vi "Run_VI_Named_specific.vi"(8 "Run VI Named String":string, 10 "Earlier Filenames":path[](array[path]), 11 "Multi Run Row":T1 {"Carrier_2 Q (l/min)" format="%#.2f"; "Row Duration (mins)" format="%#.1f"; "Row No" min=0; "Trace Gas Concentration (%)" min=0.0 format="%#_4f"; "Carrier_1 Q (l/min)" format="%#.4f"; "Start X" format="%#.2f"; "Start Y" format="%#.2f"; "Start Z" format="%#.2f"; "End X" format="%#.2f"; "End Y" format="%#.2f"; "End Z" format="%#.2f"; "Tunnel Speed" format="%#.2f"; "Averaging time (mins)" min=0.0 format="%#.2f"}) -> (0 "Scalable Time (Sec)":dbl format="%.2f", 1 "Fixed Time (Sec)":dbl format="%.2f", 2 "Channel Names":string[](array[string]), 3 "Checks":string[](array[string]), 4 "Error String":string, 5 "Check Meas Setup?":bool, 6 "Check for start NaNs?":bool)   [LabVIEW 2022 SP3]
uses:
  Gen Trav/Traverse_cluster.ctl
  Gen Trav/Spacing.ctl
  Controls/Multi_run_mode.ctl
  Globals/Preference_global.vi
  Globals/Extra_Commands_Global.vi
panel:
  # "X           Y          Z"
  # "Start"
  # "End"
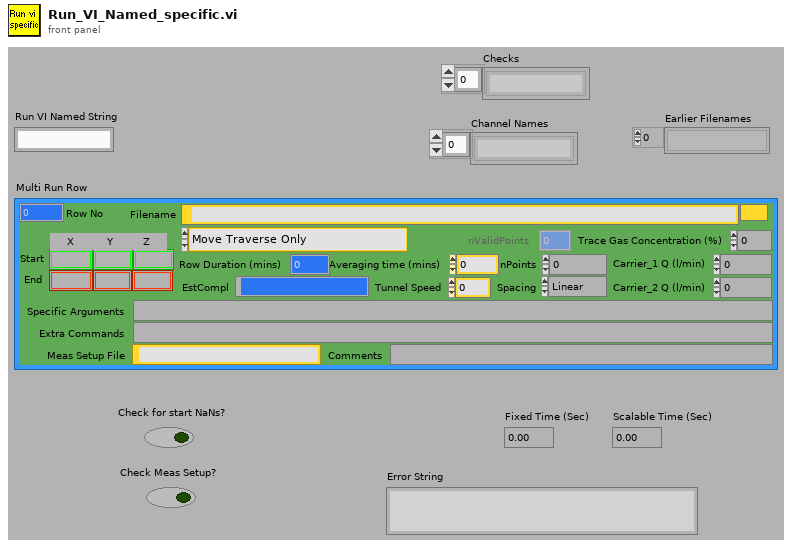
[diagram p1: front panel]
types:
  T1 = typedef "Traverse_cluster.ctl" = cluster{"Start X":sgl, "Start Y":sgl, "Start Z":sgl, "End X":sgl, "End Y":sgl, "End Z":sgl, "nPoints":i32, "Spacing":T2, "Filename":path, "Tunnel Speed":dbl, "Averaging time (mins)":dbl, "Extra Commands":string, "Carrier_1 Q (l/min)":dbl, "Carrier_2 Q (l/min)":dbl, "Trace Gas Concentration (%)":dbl, "Specific Arguments":string, "Comments":string, "Row No":i32, "Row Type Selector":T3, "EstCompl":string, "Row Duration (mins)":dbl, "nValidPoints":i32, "Meas Setup File":string}
  T2 = typedef "Spacing.ctl" = enum16{"Linear", "Log", "Gauss", "Specified", "N/A"}
  T3 = typedef "Multi_run_mode.ctl" = enum16{"Move Traverse Only", "Set Tunnel Speed Only", "Set Source Only", "Set Measurement Conditions", "Single Measurement", "Vertical Profile", "Lateral Profile", "Longitudinal Profile", "Multi-Axis Profile", "Explore Volume", "Auto Calibrate", "Meas Fast FID Bkgnd", "Check Beam Power", "Scanning Valve Measurement", "Run VI Named:", "Set ADAM Ch", "Wait (minutes)", "Send Message", "Synchronize With:", "Fall Back to this Row", "Turn Off Row Repeating", "Traverse 3D Volume", "Blank Row", "Jump to Fall Back Row"}
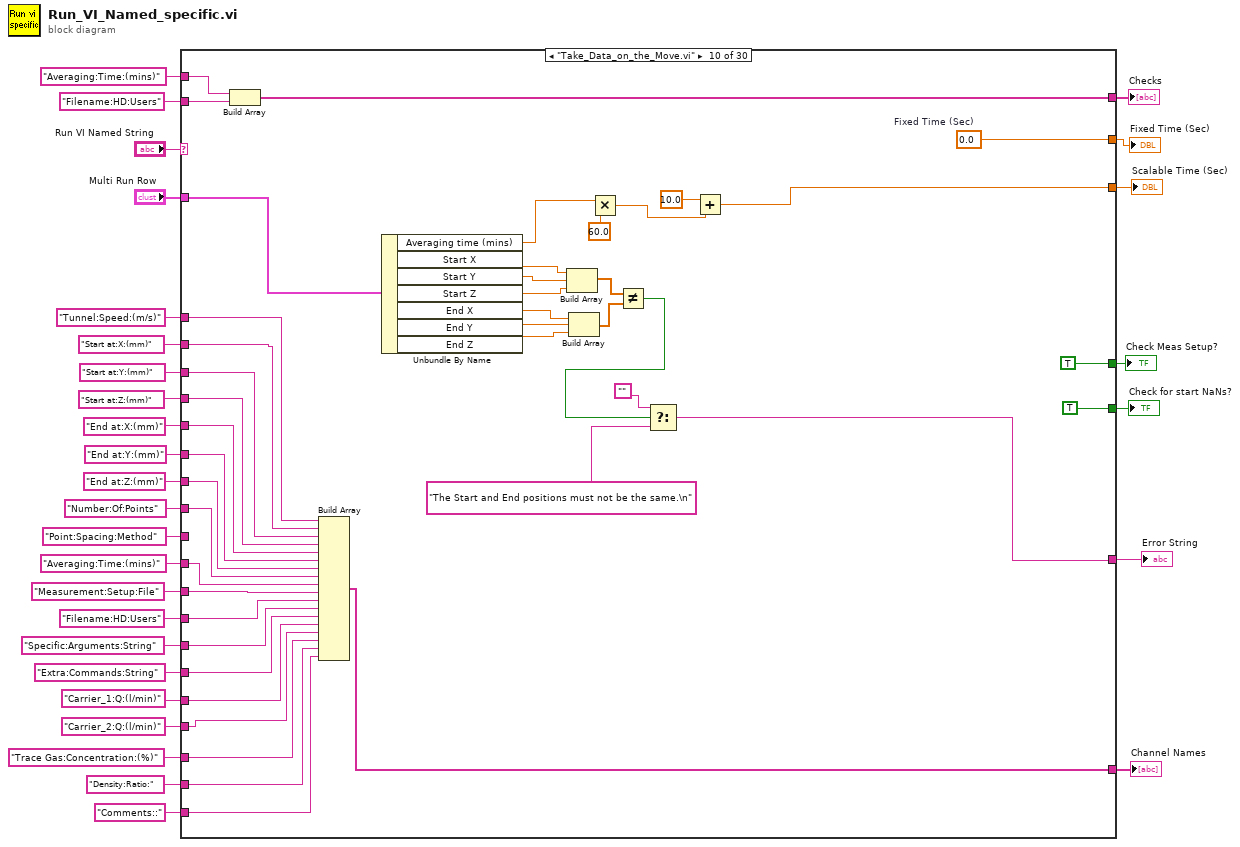
[diagram p0: block diagram]
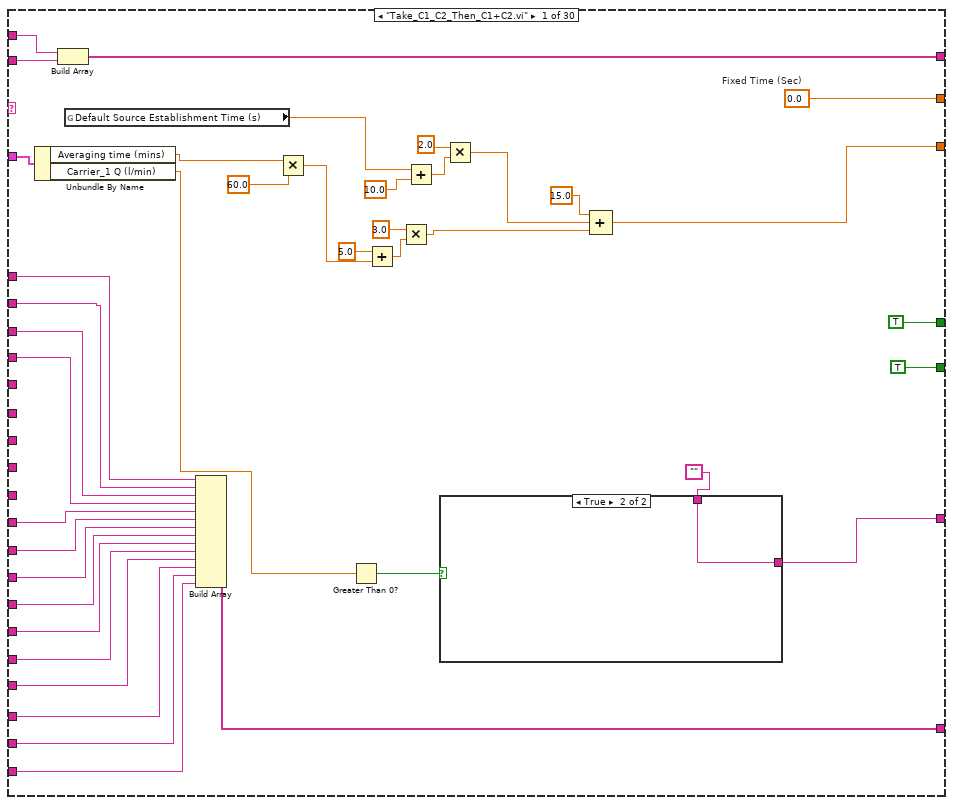
[diagram p2: hidden frame]
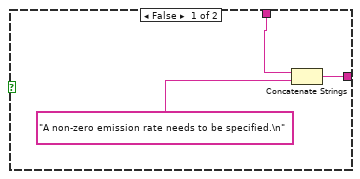
[diagram p3: hidden frame]
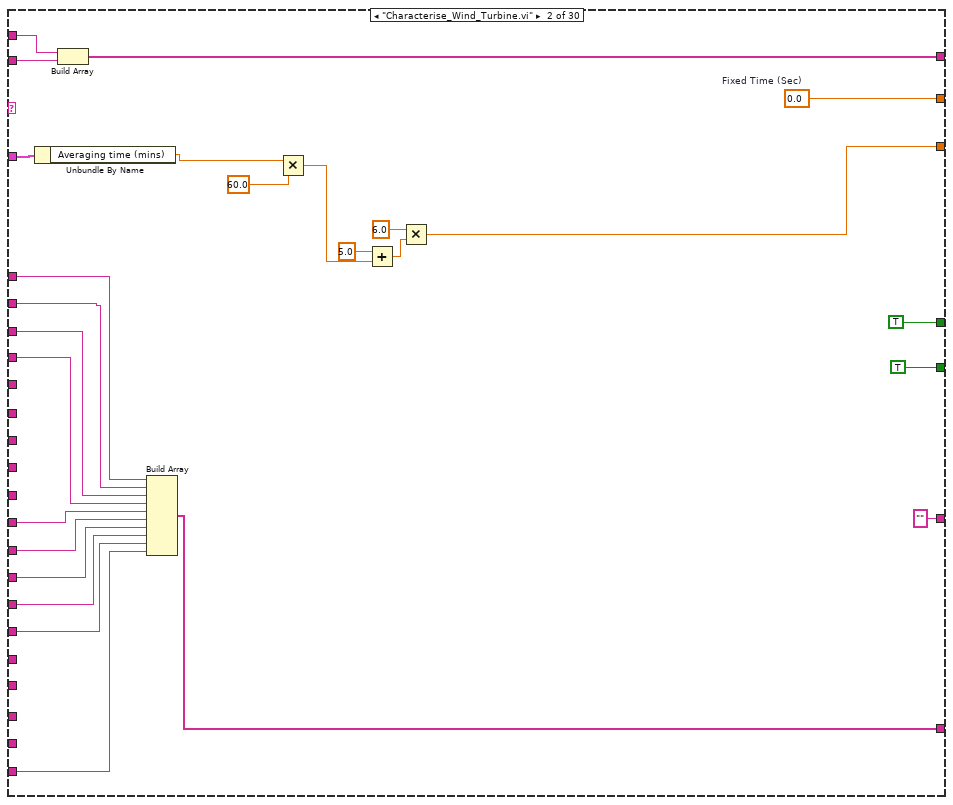
[diagram p4: hidden frame]
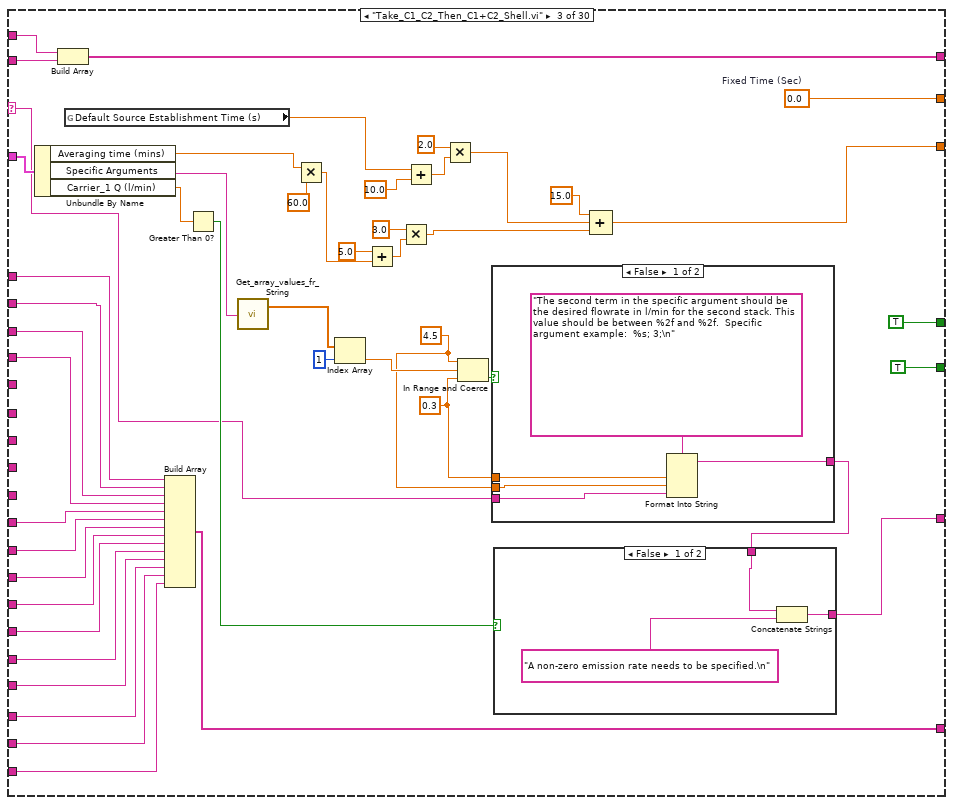
[diagram p5: hidden frame]
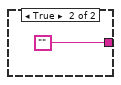
[diagram p7: hidden frame]
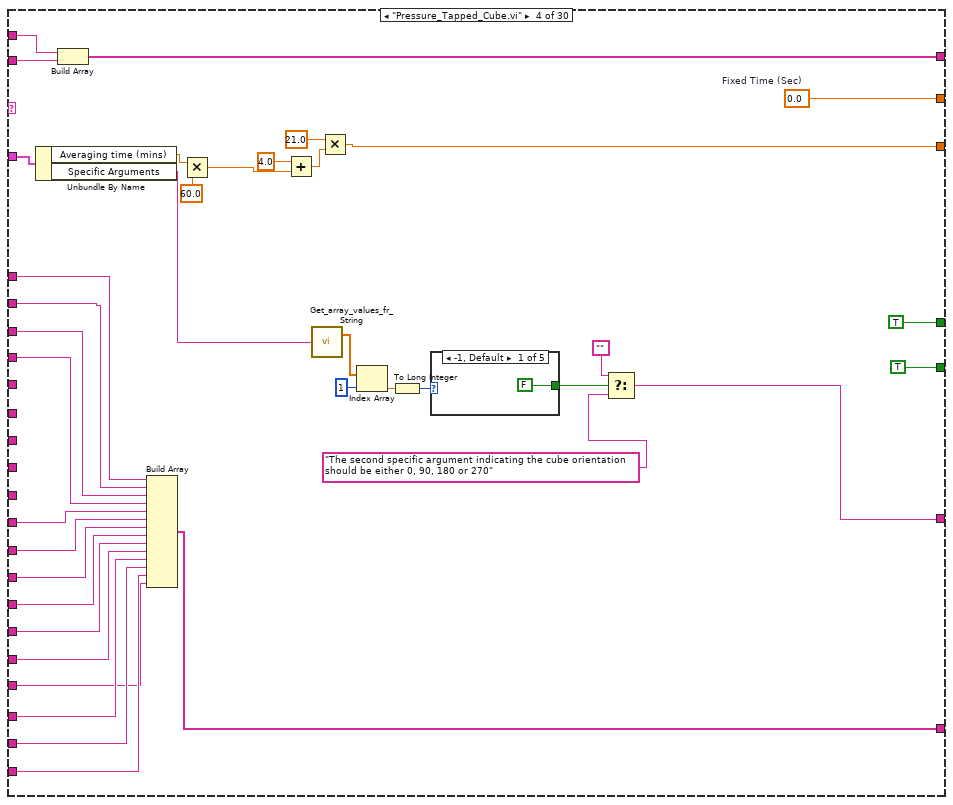
[diagram p8: hidden frame]
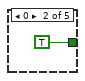
[diagram p9: hidden frame]
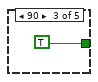
[diagram p10: hidden frame]
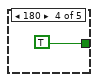
[diagram p11: hidden frame]
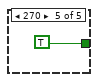
[diagram p12: hidden frame]
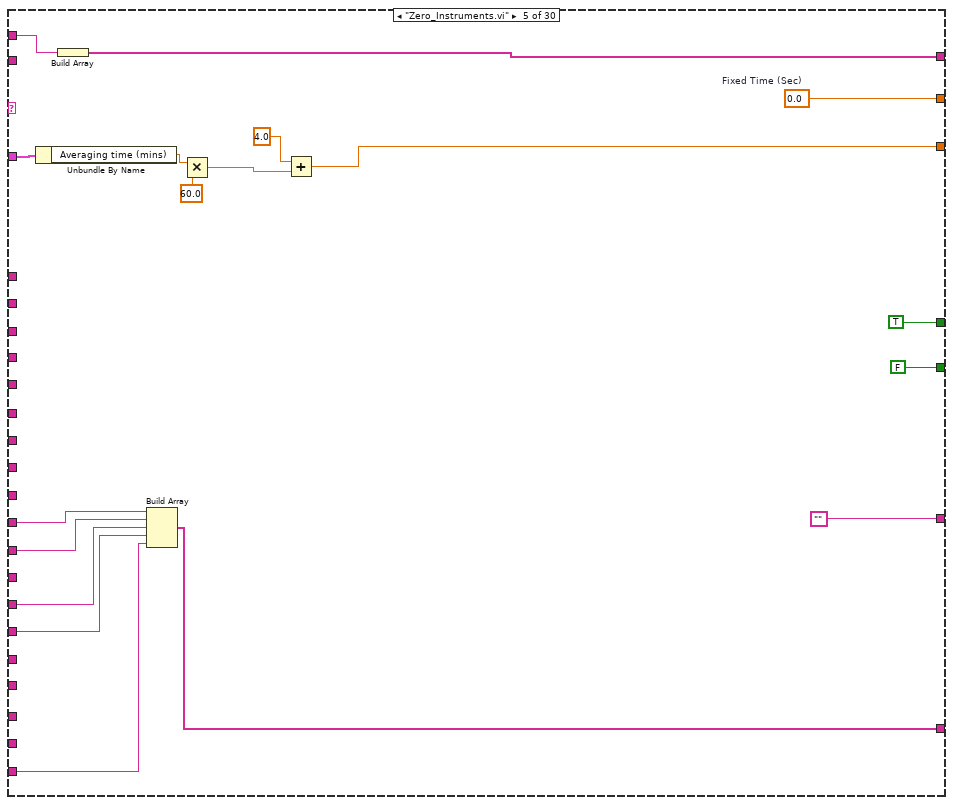
[diagram p13: hidden frame]
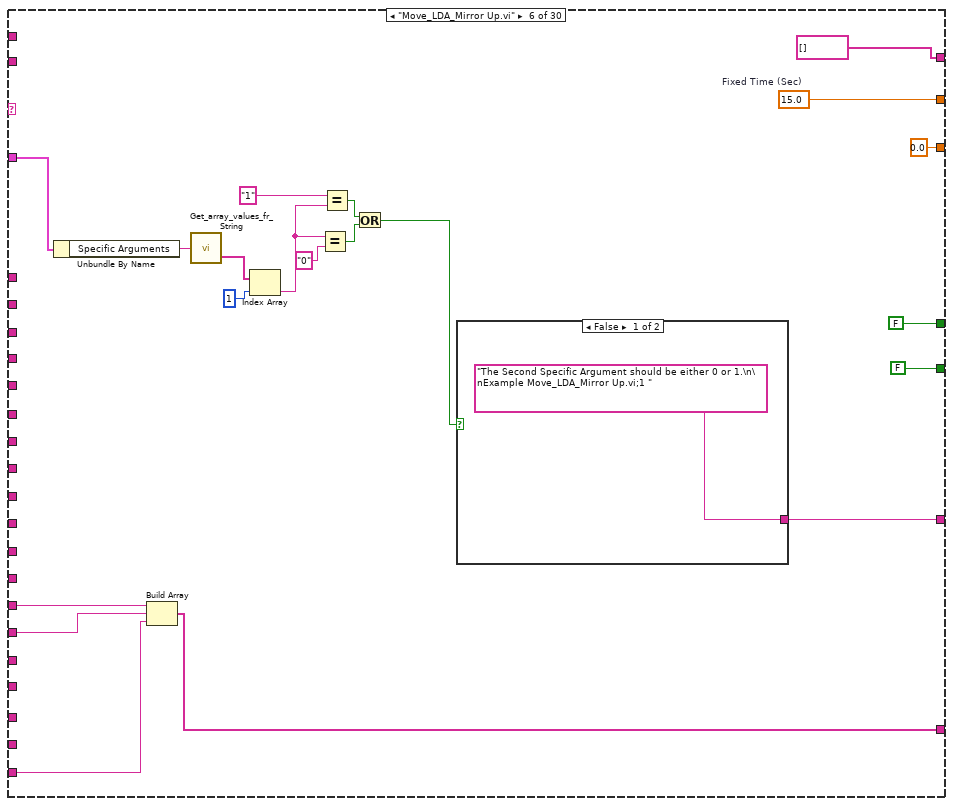
[diagram p14: hidden frame]
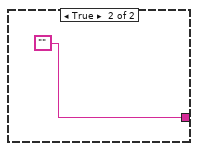
[diagram p15: hidden frame]
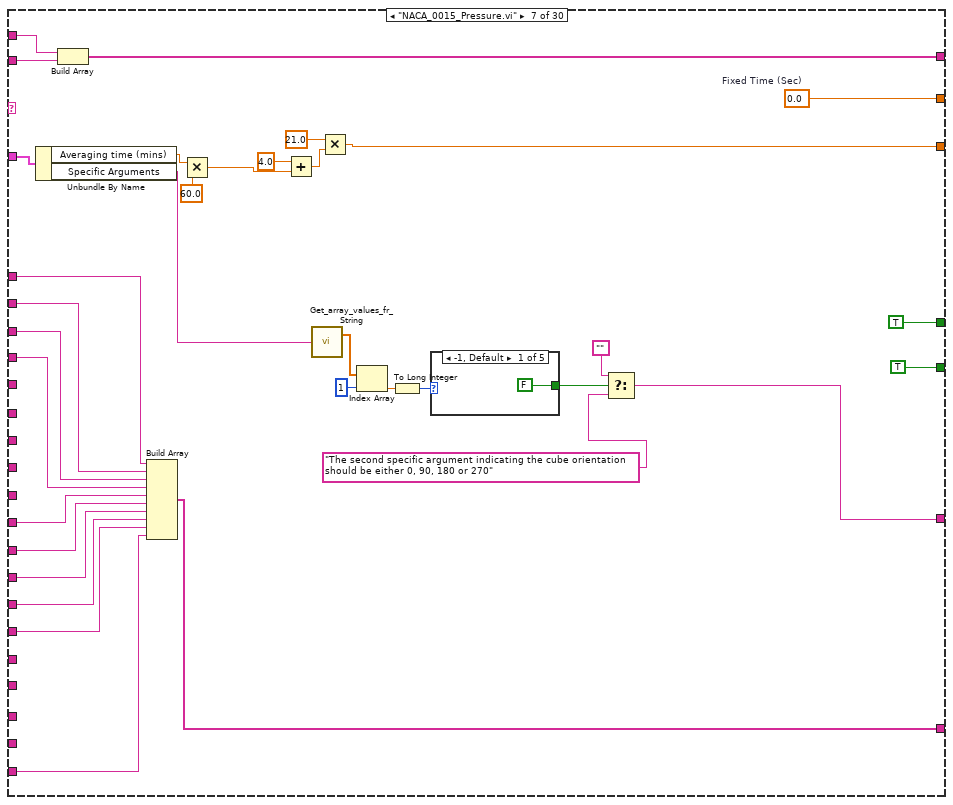
[diagram p16: hidden frame]
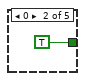
[diagram p17: hidden frame]
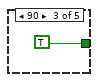
[diagram p18: hidden frame]
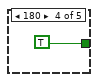
[diagram p19: hidden frame]
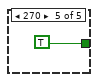
[diagram p20: hidden frame]
diagram:
  n1 = case shown="\"Take_Data_on_the_Move.vi\"" "Run VI Named String" {
    selector: "Run VI Named String" -> [_ _ w103 _ _ _ _ _ _ _ _ _ _ _ _ _ _ _ _ _ _ _ _ _ _ _ _ _ _ _]
    tunnel: "Multi Run Row" -> [w70 w100 w148 w196 w219 w224 w275 w315 w358 w368 _ w422 _ _ _ w500 _ _ w540 _ _ w580 w615 w640 w663 _ _ w741 w769 w801]
    tunnel: [w69 w99 w147 w195 w218 w239 w274 w314 w357 w401 w417 w432 0.0 ("Fixed Time (Sec)") 0.0 ("Fixed Time (Sec)") 5.0 ("Fixed Time (Sec)") 5.0 ("Fixed Time (Sec)") 5.0 ("Fixed Time (Sec)") 5.0 ("Fixed Time (Sec)") 5.0 ("Fixed Time (Sec)") 5.0 ("Fixed Time (Sec)") 5.0 ("Fixed Time (Sec)") 5.0 ("Fixed Time (Sec)") 5.0 ("Fixed Time (Sec)") 5.0 ("Fixed Time (Sec)") 30.0 ("Fixed Time (Sec)") 40.0 ("Fixed Time (Sec)") w709 w733 w768 w800] -> w29
    tunnel: [w55 w76 w133 w169 w202 0.0 ("value") w254 w294 w339 w366 60.0 ("value") 0.0 ("value") 6.0 ("value") 6.0 ("value") 0.0 ("value") 0.0 ("value") 0.0 ("value") 0.0 ("value") w535 0.0 ("value") 0.0 ("value") 0.0 ("value") 0.0 ("value") 0.0 ("value") 270.0 ("value") 0.0 ("value") w710 w740 40.0 ("value") 30.0 ("value")] -> w28
    tunnel: "Averaging:Time:(mins)" ("Label for value") -> [w54 w92 w132 w192 w215 _ w271 w311 w354 w399 w416 _ _ _ _ _ _ _ w543 _ _ _ _ _ _ _ _ _ _ _]
    tunnel: "Filename:HD:Users" ("Label for value") -> [w53 w91 w131 w191 _ _ w270 w310 w353 w398 w415 _ _ _ _ _ _ w524 w541 _ _ _ _ _ _ _ _ _ _ w778]
    tunnel: [TRUE TRUE TRUE TRUE FALSE FALSE TRUE TRUE FALSE TRUE TRUE FALSE FALSE FALSE FALSE FALSE FALSE FALSE FALSE FALSE FALSE FALSE FALSE FALSE FALSE FALSE FALSE FALSE TRUE TRUE] -> w25
    tunnel: [TRUE TRUE TRUE TRUE TRUE FALSE TRUE TRUE TRUE TRUE TRUE FALSE FALSE FALSE FALSE FALSE FALSE TRUE TRUE FALSE FALSE FALSE FALSE FALSE FALSE FALSE FALSE TRUE FALSE TRUE] -> w24
    tunnel: [w50 w88 w128 w188 w212 string[] [] w267 w307 w350 w395 w412 string[] [] string[] [] string[] [] string[] [] string[] [] string[] [] string[] [] w542 string[] [] string[] [] string[] [] string[] [] string[] [] string[] [] string[] [] string[] [] string[] [] string[] [] w777] -> w23
    tunnel: "Tunnel:Speed:(m/s)" ("Label for value") -> [w49 w87 w127 w187 _ _ w244 w284 _ w394 _ w423 w447 w473 _ _ _ _ _ _ _ _ _ _ _ _ _ w720 _ _]
    tunnel: "Start at:X:(mm)" ("Label for value") -> [w48 w86 w126 w186 _ _ w243 w283 _ w393 w411 _ w456 w477 _ _ w515 _ _ _ _ _ w614 w647 w671 w691 _ _ w765 w797]
    tunnel: "Start at:Y:(mm)" ("Label for value") -> [w47 w85 w125 w185 _ _ w242 w282 _ w392 w410 _ w455 w476 _ _ _ _ _ _ _ _ w613 _ _ w694 _ _ w764 w796]
    tunnel: "Start at:Z:(mm)" ("Label for value") -> [w46 w84 w124 w184 _ _ w266 w306 _ w391 w409 _ w454 w475 _ _ _ _ _ _ _ _ w612 _ _ _ _ _ w763 w795]
    tunnel: "Averaging:Time:(mins)" ("Label for value") -> [w45 w83 w123 w183 w211 _ w265 w305 w335 w390 _ _ w446 w472 _ _ _ _ w545 _ _ _ _ _ _ _ _ w729 _ _]
    tunnel: "Measurement:Setup:File" ("Label for value") -> [w44 w82 w122 w182 w210 _ w264 w304 w349 w389 w408 _ w442 w468 _ _ _ w526 w546 _ _ _ w609 w644 w667 w695 _ w730 _ w779]
    tunnel: "Filename:HD:Users" ("Label for value") -> [w43 w81 w121 w181 _ _ w263 w303 w348 w388 _ _ w448 w474 _ _ _ _ w544 _ _ w581 w610 w645 _ _ _ w731 _ w776]
    tunnel: "Specific:Arguments:String" ("Label for value") -> [w42 w80 w120 w180 w209 w235 w262 w302 w347 w387 w407 w429 w441 w467 w491 w511 w521 w532 w552 w562 w572 w588 w611 w646 w668 w696 w717 w732 w756 w775]
    tunnel: "Extra:Commands:String" ("Label for value") -> [w41 w79 w119 w179 w208 w231 w261 w301 w346 w386 w406 w428 w440 w466 w490 w510 _ _ w551 w561 w571 w587 w622 w655 w669 w697 w716 w745 w757 w791]
    tunnel: "Carrier_1:Q:(l/min)" ("Label for value") -> [w31 _ w101 w178 _ _ _ _ _ w385 _ _ w445 w471 _ _ _ _ _ _ _ _ _ _ _ _ _ _ _ _]
    tunnel: "Trace Gas:Concentration:(%)" ("Label for value") -> [w40 _ w118 w177 _ _ _ _ _ w361 _ _ w444 w470 _ _ _ _ _ _ _ _ _ _ _ _ _ _ _ _]
    tunnel: "Density:Ratio:" ("Label for value") -> [w39 _ w117 w176 _ _ _ _ _ w384 _ _ w443 w469 _ _ _ _ _ _ _ _ _ _ _ _ _ _ _ _]
    tunnel: "Comments::" ("Label for value") -> [w38 w78 w116 w175 w204 w232 w260 w300 w345 w383 w405 w427 w439 w465 w489 w509 w520 w531 w550 w560 w570 w586 w621 w654 w670 w698 w715 w744 w760 w792]
    tunnel: [w37 w77 w115 w174 w207 w236 w259 w299 w344 w382 w404 w426 w438 w464 w488 w508 w519 w530 w549 w559 w569 w585 w620 w653 w675 w703 w714 w743 w762 w794] -> w10
    tunnel: [w35 "" ("Error Comments") w104 w160 "" w220 w245 w285 w337 w365 "" w418 "" "" "" w494 "" "" "" "" "" w576 w599 "" w660 "" "" w735 w759 w780] -> w3
    tunnel: "End at:X:(mm)" ("Label for value") -> [_ _ _ _ _ _ _ _ _ w364 _ _ w453 _ _ _ _ _ _ _ _ _ _ _ _ w693 _ _ _ w793]
    tunnel: "End at:Y:(mm)" ("Label for value") -> [_ _ _ _ _ _ _ _ _ w363 _ _ w452 _ _ _ _ _ _ _ _ _ _ _ _ w692 _ _ _ _]
    tunnel: "End at:Z:(mm)" ("Label for value") -> [_ _ _ _ _ _ _ _ _ w362 _ _ w451 _ _ _ _ _ _ _ _ _ _ _ _ _ _ _ _ _]
    tunnel: "Number:Of:Points" ("Label for value") -> [_ _ _ _ _ _ _ w281 w336 w359 _ _ w450 _ _ _ _ _ _ _ _ _ _ _ _ _ _ _ _ _]
    tunnel: "Point:Spacing:Method" ("Label for value") -> [_ _ _ _ _ _ _ _ w334 _ _ _ w449 _ _ _ _ _ _ _ _ _ _ _ _ _ _ _ _ _]
    tunnel: "Carrier_2:Q:(l/min)" ("Label for value") -> [w32 _ w102 w159 _ _ _ _ _ w360 _ _ w437 w463 _ _ _ _ _ _ _ _ _ _ _ _ _ _ _ _]
    frame "Take_C1_C2_Then_C1+C2.vi" {
      w69 = 0.0  # Fixed Time (Sec)
      n2 = Unbundle By Name(w70) -> ("Averaging time (mins)"=w58:dbl, "Carrier_1 Q (l/min)"=w34:dbl)
      n3 = Build Array(w54, w53) -> (w50:string[])
      n4 = global read "Preference_global.vi" "Default Source Establishment Time (s)"() -> (w59:dbl)
      n5 = Build Array(w49, w48, w47, w46, w45, w44, w43, w42, w41, w31, w32, w40, w39, w38) -> (w37:string[])
      n6 = Multiply(x=w58, y=60.0) -> (x*y=w56:dbl)
      n7 = Greater Than 0?(x=w34) -> (x > 0?=w33:bool)
      n8 = Add(x=5.0, y=w56) -> (x+y=w62:dbl)
      n9 = Multiply(x=3.0, y=w62) -> (x*y=w66:dbl)
      n10 = Add(x=w59, y=10.0) -> (x+y=w64:dbl)
      n11 = case shown="True" w33 {
        tunnel: "" -> [w72 w74]
        tunnel: [w71 w74] -> w35
        frame False {
          n12 = Concatenate Strings(w72, "A non-zero emission rate needs to be specified.\n") -> (w71:string)
        }
        frame True {
        }
      }
      n13 = Multiply(x=2.0, y=w64) -> (x*y=w67:dbl)
      n14 = Compound Arithmetic op=ADD(15.0 ("value"), w67, w66) -> (w55:dbl)
    }
    frame "Characterise_Wind_Turbine.vi" {
      w99 = 0.0  # Fixed Time (Sec)
      n15 = Unbundle By Name(w100) -> ("Averaging time (mins)"=w95:dbl)
      n16 = Build Array(w92, w91) -> (w88:string[])
      n17 = Build Array(w87, w86, w85, w84, w83, w82, w81, w80, w79, w78) -> (w77:string[])
      n18 = Multiply(x=w95, y=60.0) -> (x*y=w93:dbl)
      n19 = Add(x=5.0, y=w93) -> (x+y=w98:dbl)
      n20 = Multiply(x=6.0, y=w98) -> (x*y=w76:dbl)
    }
    frame "Take_C1_C2_Then_C1+C2_Shell.vi" {
      w108 = 4.5 ("upper limit")
      w109 = 0.3 ("lower limit")
      w147 = 0.0  # Fixed Time (Sec)
      n21 = Unbundle By Name(w148) -> ("Averaging time (mins)"=w136:dbl, "Specific Arguments"=w112:string, "Carrier_1 Q (l/min)"=w107:dbl)
      n22 = Build Array(w132, w131) -> (w128:string[])
      n23 = global read "Preference_global.vi" "Default Source Establishment Time (s)"() -> (w137:dbl)
      n24 = Build Array(w127, w126, w125, w124, w123, w122, w121, w120, w119, w101, w102, w118, w117, w116) -> (w115:string[])
      n25 = Greater Than 0?(x=w107) -> (x > 0?=w106:bool)
      n26 = call "Get_array_values_fr_String.vi"("String Value"=w112) -> ("Numeric Array"=w114:dbl[])  [unwired: 1 out]
      n27 = Multiply(x=w136, y=60.0) -> (x*y=w134:dbl)
      n28 = Index Array(array=w114, index=1) -> (element=w111:dbl)
      n29 = Add(x=5.0, y=w134) -> (x+y=w140:dbl)
      n30 = Multiply(x=3.0, y=w140) -> (x*y=w144:dbl)
      n31 = Add(x=w137, y=10.0) -> (x+y=w142:dbl)
      n32 = Multiply(x=2.0, y=w142) -> (x*y=w145:dbl)
      n33 = In Range and Coerce(upper limit=w108, x=w111, lower limit=w109) -> (In Range?=w110:bool)  [unwired: 1 out]
      n34 = case shown="False" w110 {
        tunnel: [w153 ""] -> w105
        tunnel: w103 -> [w157 _]
        tunnel: w109 -> [w156 _]
        tunnel: w108 -> [w155 _]
        frame False {
          n35 = Format Into String(format string="The second term in the specific argument should be the desired flowrate in l/min for the second stack. This value should be between %2f and %2f.  Specific argument example:  %s; 3;\n", w156, w155, w157) -> (resulting string=w153:string)  [unwired: 2 in, 1 out]
        }
        frame True {
        }
      }
      n36 = case shown="False" w106 {
        tunnel: w105 -> [w150 w152]
        tunnel: [w149 w152] -> w104
        frame False {
          n37 = Concatenate Strings(w150, "A non-zero emission rate needs to be specified.\n") -> (w149:string)
        }
        frame True {
        }
      }
      n38 = Compound Arithmetic op=ADD(15.0 ("value"), w145, w144) -> (w133:dbl)
    }
    frame "Pressure_Tapped_Cube.vi" {
      w195 = 0.0  # Fixed Time (Sec)
      n39 = Unbundle By Name(w196) -> ("Averaging time (mins)"=w194:dbl, "Specific Arguments"=w161:string)
      n40 = Build Array(w192, w191) -> (w188:string[])
      n41 = Build Array(w187, w186, w185, w184, w183, w182, w181, w180, w179, w178, w177, w176, w175, w159) -> (w174:string[])
      n42 = Multiply(x=w194, y=60.0) -> (x*y=w170:dbl)
      n43 = Add(x=4.0, y=w170) -> (x+y=w173:dbl)
      n44 = call "Get_array_values_fr_String.vi"("String Value"=w161) -> ("Numeric Array"=w163:dbl[])  [unwired: 1 out]
      n45 = Multiply(x=21.0, y=w173) -> (x*y=w169:dbl)
      n46 = Index Array(array=w163, index=1) -> (element=w164:dbl)
      n47 = To Long Integer(number=w164) -> (32bit integer=w165:i32)
      n48 = case shown="-1, Default" w165 {
        tunnel: [FALSE TRUE TRUE TRUE TRUE] -> w168
        frame -1, Default {
        }
        frame 0 {
        }
        frame 90 {
        }
        frame 180 {
        }
        frame 270 {
        }
      }
      n49 = Select(t="", s=w168, f="The second specific argument indicating the cube orientation should be either 0, 90, 180 or 270") -> (s? t:f=w160:string)
    }
    frame "Zero_Instruments.vi" {
      w218 = 0.0  # Fixed Time (Sec)
      n50 = Unbundle By Name(w219) -> ("Averaging time (mins)"=w217:dbl)
      n51 = Build Array(w215) -> (w212:string[])
      n52 = Build Array(w211, w210, w209, w208, w204) -> (w207:string[])
      n53 = Multiply(x=w217, y=60.0) -> (x*y=w205:dbl)
      n54 = Add(x=4.0, y=w205) -> (x+y=w202:dbl)
    }
    frame "Move_LDA_Mirror Up.vi" {
      w239 = 15.0  # Fixed Time (Sec)
      n55 = Unbundle By Name(w224) -> ("Specific Arguments"=w225:string)
      n56 = Build Array(w235, w231, w232) -> (w236:string[])
      n57 = call "Get_array_values_fr_String.vi"("String Value"=w225) -> ("String array"=w227:string[])  [unwired: 1 out]
      n58 = Index Array(array=w227, index=1) -> (element=w229:string)
      n59 = Equal?(x=w229, y="0") -> (x = y?=w222:bool)
      n60 = Equal?(x="1" ("String to match"), y=w229) -> (x = y?=w223:bool)
      n61 = Or(x=w223, y=w222) -> (x .or. y?=w221:bool)
      n62 = case shown="False" w221 {
        tunnel: ["The Second Specific Argument should be either 0 or 1.\n\nExample Move_LDA_Mirror Up.vi;1 " ""] -> w220
        frame False {
        }
        frame True {
        }
      }
    }
    frame "NACA_0015_Pressure.vi" {
      w274 = 0.0  # Fixed Time (Sec)
      n63 = Unbundle By Name(w275) -> ("Averaging time (mins)"=w273:dbl, "Specific Arguments"=w246:string)
      n64 = Build Array(w271, w270) -> (w267:string[])
      n65 = Build Array(w244, w243, w242, w266, w265, w264, w263, w262, w261, w260) -> (w259:string[])
      n66 = Multiply(x=w273, y=60.0) -> (x*y=w255:dbl)
      n67 = Add(x=4.0, y=w255) -> (x+y=w258:dbl)
      n68 = call "Get_array_values_fr_String.vi"("String Value"=w246) -> ("Numeric Array"=w248:dbl[])  [unwired: 1 out]
      n69 = Multiply(x=21.0, y=w258) -> (x*y=w254:dbl)
      n70 = Index Array(array=w248, index=1) -> (element=w249:dbl)
      n71 = To Long Integer(number=w249) -> (32bit integer=w250:i32)
      n72 = case shown="-1, Default" w250 {
        tunnel: [FALSE TRUE TRUE TRUE TRUE] -> w253
        frame -1, Default {
        }
        frame 0 {
        }
        frame 90 {
        }
        frame 180 {
        }
        frame 270 {
        }
      }
      n73 = Select(t="", s=w253, f="The second specific argument indicating the cube orientation should be either 0, 90, 180 or 270") -> (s? t:f=w245:string)
    }
    frame "NACA_0015_Pressure_with_profile.vi" {
      w314 = 0.0  # Fixed Time (Sec)
      n74 = Unbundle By Name(w315) -> ("Averaging time (mins)"=w313:dbl, "Specific Arguments"=w286:string)
      n75 = Build Array(w311, w310) -> (w307:string[])
      n76 = Build Array(w284, w283, w282, w306, w281, w305, w304, w303, w302, w301, w300) -> (w299:string[])
      n77 = Multiply(x=w313, y=60.0) -> (x*y=w295:dbl)
      n78 = Add(x=4.0, y=w295) -> (x+y=w298:dbl)
      n79 = call "Get_array_values_fr_String.vi"("String Value"=w286) -> ("Numeric Array"=w288:dbl[])  [unwired: 1 out]
      n80 = Multiply(x=21.0, y=w298) -> (x*y=w294:dbl)
      n81 = Index Array(array=w288, index=1) -> (element=w289:dbl)
      n82 = To Long Integer(number=w289) -> (32bit integer=w290:i32)
      n83 = case shown="-1, Default" w290 {
        tunnel: [FALSE TRUE TRUE TRUE TRUE] -> w293
        frame -1, Default {
        }
        frame 0 {
        }
        frame 90 {
        }
        frame 180 {
        }
        frame 270 {
        }
      }
      n84 = Select(t="", s=w293, f="The second specific argument indicating the cube orientation should be either 0, 90, 180 or 270") -> (s? t:f=w285:string)
    }
    frame "Measure_Synthetic_Jet.vi" {
      w357 = 0.0  # Fixed Time (Sec)
      n85 = Unbundle By Name(w358) -> ("Averaging time (mins)"=w356:dbl, "Specific Arguments"=w338:string)
      n86 = Build Array(w354, w353) -> (w350:string[])
      n87 = Build Array(w336, w334, w335, w349, w348, w347, w346, w345) -> (w344:string[])
      n88 = Multiply(x=w356, y=60.0) -> (x*y=w340:dbl)
      n89 = Add(x=4.0, y=w340) -> (x+y=w343:dbl)
      n90 = call "Get_array_values_fr_String.vi"("String Value"=w338) -> ("String array"=w333:string[])  [unwired: 1 out]
      n91 = Multiply(x=21.0, y=w343) -> (x*y=w339:dbl)
      n92 = Index Array(array=w333, index #1=1 ("index")) -> (element #1=w328:string, element #2=w326:string, element #3=w325:string, element #4=w322:string)  [unwired: 3 in]
      n93 = Empty String/Path?(string/path=w322) -> (empty?=w321:bool)
      n94 = Empty String/Path?(string/path=w326) -> (empty?=w323:bool)
      n95 = Empty String/Path?(string/path=w328) -> (empty?=w327:bool)
      n96 = Empty String/Path?(string/path=w325) -> (empty?=w324:bool)
      n97 = Compound Arithmetic op=OR(w327, w323, w324, w321) -> (w331:bool)
      n98 = Select(t="The second, third and fourth specific argument indicate the min frequency, max frequency, the number of bins to use in the phase average and the target amplitude.  Set the target optimisation target value to -1 if you do not want any optimisation. Example: Measure_Synthetic_Jet.vi; 100; 1000; 50; 0.02", s=w331, f="") -> (s? t:f=w337:string)
    }
    frame "Take_Data_on_the_Move.vi" {
      w401 = 0.0  # Fixed Time (Sec)
      n99 = Build Array(w399, w398) -> (w395:string[])
      n100 = Build Array(w394, w393, w392, w391, w364, w363, w362, w359, w390, w389, w388, w387, w386, w385, w360, w361, w384, w383) -> (w382:string[])
      n101 = Unbundle By Name(w368) -> ("Averaging time (mins)"=w367:dbl, "Start X"=w369:sgl, "Start Y"=w370:sgl, "Start Z"=w371:sgl, "End X"=w372:sgl, "End Y"=w373:sgl, "End Z"=w374:sgl)
      n102 = Build Array(w369, w370, w371) -> (w376:sgl[])
      n103 = Build Array(w372, w373, w374) -> (w375:sgl[])
      n104 = Multiply(x=w367, y=60.0) -> (x*y=w380:dbl)
      n105 = Not Equal?(x=w376, y=w375) -> (x != y?=w379:bool)
      n106 = Select(t="", s=w379, f="The Start and End positions must not be the same.\n" ("Format String")) -> (s? t:f=w365:string)
      n107 = Add(x=10.0, y=w380) -> (x+y=w366:dbl)
    }
    frame "Check_FID_Response.vi" {
      w417 = 0.0  # Fixed Time (Sec)
      n108 = Build Array(w416, w415) -> (w412:string[])
      n109 = Build Array(w411, w410, w409, w408, w407, w406, w405) -> (w404:string[])
    }
    frame "Return_EnFlo_Tunnel_to_Neutral.vi" {
      w419 = 0.4 ("y")
      w432 = 6000.0  # Fixed Time (Sec)
      n110 = Unbundle By Name(w422) -> ("Tunnel Speed"=w421:dbl)
      n111 = Build Array(w423, w429, w428, w427) -> (w426:string[])
      n112 = Greater?(x=w421, y=w419) -> (0:w420:bool)
      n113 = case shown="False" w420 {
        tunnel: w419 -> [w435 _]
        tunnel: [w433 ""] -> w418
        frame False {
          n114 = Format Into String(format string="The Tunnel speed must be greater than %.1f", w435) -> (resulting string=w433:string)  [unwired: 2 in, 1 out]
        }
        frame True {
        }
      }
    }
    frame "No Match", Default {
      n115 = Build Array(w456, w455, w454, w453, w452, w451, w450, w449, w448, w447, w446, w440, w441, w445, w444, w443, w439, w442, w437) -> (w438:string[])
    }
    frame "Measurement on Remote PC.vi" {
      n116 = Build Array(w477, w476, w475, w474, w473, w472, w466, w467, w471, w470, w469, w465, w468, w463) -> (w464:string[])
    }
    frame "Set_Wind_Turbine_Speed.vi" {
      n117 = Build Array(w491, w490, w489) -> (w488:string[])
    }
    frame "Wait till chilled water below.vi" {
      n118 = Unbundle By Name(w500) -> ("Specific Arguments"=w499:string)
      n119 = Build Array(w511, w510, w509) -> (w508:string[])
      n120 = call "Get_array_values_fr_String.vi"("String Value"=w499) -> ("Numeric Array"=w502:dbl[])  [unwired: 1 out]
      n121 = Index Array(array=w502, index=1) -> (element=w498:dbl)
      n122 = In Range and Coerce(upper limit=25.0, x=w498, lower limit=4.0) -> (In Range?=w495:bool)  [unwired: 1 out]
      n123 = Select(t="", s=w495, f="The second specific argument setting  the chilled water temperature below which the run can continue should be in the range of 4 to 25 degC.") -> (s? t:f=w494:string)
    }
    frame "CPP-MoveTT.vi" {
      # "Desired angle can now be held in X; previously passed after semicolon in Specific Arguments"
      n124 = Build Array(w515, w521, w520) -> (w519:string[])
    }
    frame "ESC Run VI Named.vi" {
      n125 = Build Array(w524, w526, w532, w531) -> (w530:string[])
    }
    frame "Capture_Flow_Vis.vi" {
      n126 = Build Array(w543, w541) -> (w542:string[])
      n127 = Unbundle By Name(w540) -> ("Averaging time (mins)"=w539:dbl)
      n128 = Build Array(w545, w546, w544, w552, w551, w550) -> (w549:string[])
      n129 = Multiply(x=60.0, y=w539) -> (x*y=w537:dbl)
      n130 = Add(x=w537, y=60.0) -> (x+y=w535:dbl)
    }
    frame "Shut_Down_A_Tunnel.vi", "Shut_down_EnFlo_Tunnel.vi" {
      n131 = Build Array(w562, w561, w560) -> (w559:string[])
    }
    frame "Post Process Files in MultiRun.vi", "Shut_Down_Aero_Tunnel.vi" {
      n132 = Build Array(w572, w571, w570) -> (w569:string[])
    }
    frame "Update_Inlet_Temp_Profile.vi" {
      n133 = Unbundle By Name(w580) -> ("Filename"=w575:path)
      n134 = Build Array(w581, w588, w587, w586) -> (w585:string[])
      n135 = Search 1D Array(1D array="Earlier Filenames", element=w575) -> (index of element=w578:i32)  [unwired: 1 in]
      n136 = case shown="0, Default" w578 {
        tunnel: w575 -> [_ w597]
        tunnel: [TRUE ("exists?") w596] -> w577
        frame 0, Default {
        }
        frame -1 {
          n137 = call "Does_file_exist_(simple).vi"("Pathname"=w597) -> ("exists?"=w596:bool)
        }
      }
      n138 = case shown="False" w577 {
        tunnel: [w591 ""] -> w576
        tunnel: w575 -> [w593 _]
        frame False {
          n139 = Format Into String(format string="Cannot find Filename%s", w593) -> (resulting string=w591:string)  [unwired: 2 in, 1 out]
        }
        frame True {
        }
      }
    }
    frame "Datum_Image_Calibration.vi" {
      n140 = Unbundle By Name(w615) -> ("Filename"=w606:path, "Specific Arguments"=w604:string)
      n141 = Build Array(w614, w613, w612, w609, w610, w611, w622, w621) -> (w620:string[])
      n142 = disable-structure shown="TARGET_TYPE==Windows" {
        disable-tunnel: [w625 _] -> w598
        frame condition #0 (active) {
          n143 = call "Get_Available_Cameras.vi"() -> ("Cameras"=w625:string[])  [unwired: 2 in, 1 out]
        }
        frame condition #1 {
        }
      }
      n144 = call "Get_array_values_fr_String.vi"("String Value"=w604) -> ("String array"=w603:string[])  [unwired: 1 out]
      n145 = call "Current_Filepath.vi"("Short_Name"="Cal" ("Data Type"), "Filename in"=w606, "Data Type"="Calibrations") -> ("Filename Out"=w605:path)  [unwired: 1 in, 1 out]
      n146 = Index Array(array=w603, index=2) -> (element=w600:string)
      n147 = call "Does_file_exist_(simple).vi"("Pathname"=w605) -> ("exists?"=w616:bool)
      n148 = case shown="False" w616 {
        tunnel: w605 -> [w638 _]
        frame False {
          n149 = call "Write Characters with check.vi"("String to Write"="Created so that multirun checker is happy that the file exists", "file (use dialog)"=w638) -> ()  [unwired: 2 in, 1 out]
        }
        frame True {
        }
      }
      n150 = Search 1D Array(1D array=w598, element=w600) -> (index of element=w601:i32)  [unwired: 1 in]
      n151 = case shown="-1" w601 {
        tunnel: w600 -> [_ w632]
        tunnel: ["" w630] -> w599
        tunnel: w598 -> [_ w629]
        frame Default {
        }
        frame -1 {
          n152 = for {
            shift-right: [w636] -> w627
            shift-left: "" -> [w635]
            tunnel: w629 -> [w634] mode=indexing
            n153 = Concatenate Strings(w635, w634, "\r\n") -> (w636:string)
          }
          n154 = Format Into String(format string="\"%s\" is not a valid Camera Name.\nThe 3rd Specific Argument should be a valid Camera Name.\nValid Camera Names are:\n%s", w632, w627) -> (resulting string=w630:string)  [unwired: 2 in, 1 out]
        }
      }
    }
    frame "Datum_Turntable_Image.vi" {
      n155 = Unbundle By Name(w640) -> ("Filename"=w641:path)
      n156 = Build Array(w647, w644, w645, w646, w655, w654) -> (w653:string[])
      n157 = call "Current_Filepath.vi"("Short_Name"="Cal" ("Data Type"), "Filename in"=w641, "Data Type"="Calibrations") -> ("Filename Out"=w639:path)  [unwired: 1 in, 1 out]
      n158 = call "Does_file_exist_(simple).vi"("Pathname"=w639) -> ("exists?"=w648:bool)
      n159 = case shown="False" w648 {
        tunnel: w639 -> [w659 _]
        frame False {
          n160 = call "Write Characters with check.vi"("String to Write"="Created so that multirun checker is happy that the file exists", "file (use dialog)"=w659) -> ()  [unwired: 2 in, 1 out]
        }
        frame True {
        }
      }
    }
    frame "EnFlo_Turntable_Control.vi" {
      n161 = Unbundle By Name(w663) -> ("Extra Commands"=w662:string)
      n162 = global read "Extra_Commands_Global.vi" "Datum Image"() -> (w664:string)
      n163 = Build Array(w671, w667, w668, w669, w670) -> (w675:string[])
      n164 = call "Extra_Commands.vi"("String to Search"=w662, "Command"=w664) -> ("String Value"=w666:string, "Command Found"=w665:bool)  [unwired: 2 in, 2 out]
      n165 = case shown="True" w665 {
        tunnel: w666 -> [_ w685]
        tunnel: ["" w683] -> w661
        frame False {
        }
        frame True {
          n166 = call "Get_array_values_fr_String.vi"("String Value"=w685) -> ("String array"=w686:string[])  [unwired: 1 out]
          n167 = Index Array(array=w686) -> (element=w684:string)  [unwired: 1 in]
          n168 = Build Path(base path=path "hello", name or relative path=w684) -> (appended path=w687:path)
          n169 = call "Current_Filepath.vi"("Short_Name"="Cal" ("Data Type"), "Filename in"=w687, "Data Type"="Calibrations") -> ("Filename Out"=w682:path)  [unwired: 1 in, 1 out]
          n170 = call "Read Characters with check.vi"("file (use dialog)"=w682) -> ("Read String"=w681:string)  [unwired: 1 in, 1 out]
          n171 = call "Image_Pro_controls_from_string.vi"("Setup String"=w681) -> ("Camera"=w683:string)  [unwired: 6 in, 4 out]
        }
      }
      n172 = case shown="\"False\", Default" w661 {
        tunnel: ["\"TurnTable_Cam\" has not been selected." ""] -> w660
        frame "False", Default {
        }
        frame "TurnTable_Cam" {
        }
      }
    }
    frame "Plot_Rectangle.vi" {
      n173 = Build Array(w691, w694, w693, w692, w695, w696, w697, w698) -> (w703:string[])
    }
    frame "Find_Beam_Max_Pos.vi" {
      w712 = 240.0  # Fixed Time (Sec)
      w710 = 0.0  # Scalable Time (Sec)
      n174 = call "Beam_Check_Positions.vi"("Load From File?"=TRUE) -> ("Beam Names"=w707:string[])  [unwired: 6 in, 8 out]
      n175 = Build Array(w717, w716, w715) -> (w714:string[])
      n176 = Array Size(array=w707) -> (size(s)=w711:i32)
      n177 = Multiply(x=w712, y=w711) -> (x*y=w709:dbl)
    }
    frame "Find_Max_Value.vi" {
      w733 = 240.0  # Fixed Time (Sec)
      w740 = 0.0  # Scalable Time (Sec)
      n178 = Unbundle By Name(w741) -> ("Specific Arguments"=w738:string)
      n179 = Build Array(w720, w729, w730, w731, w732, w745, w744) -> (w743:string[])
      n180 = call "Get_array_values_fr_String.vi"("String Value"=w738) -> ("String array"=w739:string[])  [unwired: 1 out]
      n181 = Index Array(array=w739) -> (element #2=w737:string, element #3=w728:string, element #4=w722:string, element #5=w721:string)  [unwired: 5 in, 1 out]
      n182 = Empty String/Path?(string/path=w721) -> (empty?=w724:bool)
      n183 = Empty String/Path?(string/path=w737) -> (empty?=w727:bool)
      n184 = Empty String/Path?(string/path=w728) -> (empty?=w726:bool)
      n185 = Empty String/Path?(string/path=w722) -> (empty?=w723:bool)
      n186 = Compound Arithmetic op=OR(w727, w726, w723, w724) -> (w725:bool)
      n187 = Select(t="The second argument should be contain the fixed axis, followed by the search step in mm, the measurement channel to use for the survey and finally the data type you would like to measure, for example: Z Axis; 0.75; 2; uw/u'w'", s=w725, f="" ("Error Comments")) -> (s? t:f=w735:string)
    }
    frame "Check and Tweak Position.vi" {
      w768 = 0.0  # Fixed Time (Sec)
      n188 = Unbundle By Name(w769) -> ("Start X"=w755:sgl, "Start Y"=w754:sgl, "Start Z"=w753:sgl)
      n189 = Build Array(w755, w754, w753) -> (w752:sgl[])
      n190 = Build Array(w765, w764, w763, w756, w757, w760) -> (w762:string[])
      n191 = Not A Number/Path/Refnum?(number/path/refnum=w752) -> (NaN/Path/Refnum?=w751:bool[])
      n192 = Or Array Elements(Boolean array=w751) -> (logical OR=w750:bool)
      n193 = Select(t="Start X Y Z must be valid numbers.", s=w750, f="") -> (s? t:f=w759:string)
    }
    frame "Get 3D Live Position Offset.vi" {
      w800 = 5.0  # Fixed Time (Sec)
      n194 = Unbundle By Name(w801) -> ("Specific Arguments"=w787:string)
      n195 = Build Array(w778) -> (w777:string[])
      n196 = Build Array(w797, w796, w795, w793, w779, w776, w775, w791, w792) -> (w794:string[])
      n197 = call "Get_array_values_fr_String.vi"("String Value"=w787) -> ("Numeric Array"=w786:dbl[])  [unwired: 1 out]
      n198 = Array Subset(array=w786, index=1, length=1) -> (w783:dbl[])
      n199 = Array Size(array=w786) -> (size(s)=w785:i32)
      n200 = Not A Number/Path/Refnum?(number/path/refnum=w783) -> (NaN/Path/Refnum?=w773:bool[])
      n201 = Not(x=w773) -> (.not. x?=w772:bool[])
      n202 = Equal?(x=w785, y=2) -> (x = y?=w782:bool)
      n203 = And Array Elements(Boolean array=w772) -> (logical AND=w771:bool)
      n204 = Compound Arithmetic op=AND(w782, w771) -> (w781:bool)
      n205 = Select(t="", s=w781, f="Example Specific Argument\nGet 3D Live Position Offset.vi; Datum value that you wish to take away the measured height from.") -> (s? t:f=w780:string)
    }
  }
  "Fixed Time (Sec)" <- w29
  "Scalable Time (Sec)" <- w28
  "Check Meas Setup?" <- w24
  "Error String" <- w3
  "Check for start NaNs?" <- w25
  "Checks" <- w23
  "Channel Names" <- w10
